vi "Read Voltage.vi"(8 "error in":errorcluster, 11 "Voltmeter CFG in":refnum<class "Voltmeter CFG.lvclass">) -> (0 "error out":errorcluster, 2 "Voltage":dbl format="%#_g V", 3 "Voltmeter CFG out":refnum<class "Voltmeter CFG.lvclass">)   [LabVIEW 2023, in "OWON SDS1022.lvlib" / "Voltmeter CFG.lvclass"]
uses:
  Voltmeter CFG.lvclass
  HAL/Scope VISA/Configuration/Scope VISA CFG.lvclass/Scope VISA CFG.ctl
  Voltmeter CFG.lvclass/Voltmeter CFG.ctl
  <vilib>/Analysis/baseanly.llb/Mean (DBL).vi
  <vilib>/Analysis/NI_AALBase.lvlib
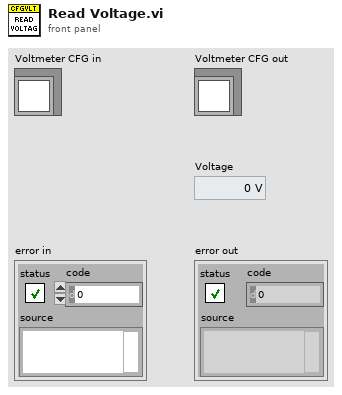
[diagram p1: front panel]
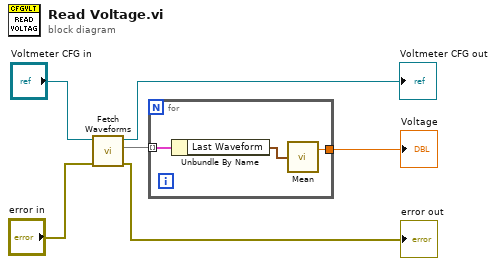
[diagram p0: block diagram]
diagram:
  n1 = call-dynamic "Fetch Waveforms.vi"("error in"="error in", "Fetch Display CFG in"="Voltmeter CFG in") -> ("error out"=→"error out":errorcluster, "Last Waveforms"=w3:map{u8, waveform(dbl)}, "Fetch Display out"=→"Voltmeter CFG out":refnum<class "Voltmeter CFG.lvclass">)  [unwired: 7 in]
  n2 = for {
    tunnel: w3 -> [w8] mode=indexing
    tunnel: [w9] -> w2
    n3 = Unbundle By Name(w8) -> ("Last Waveform"=w7:waveform(dbl))
    n4 = call-poly <vilib>:"Mean.vi"("X"=w7) -> ("mean"=w9:dbl)  [unwired: 1 out]
  }
  "Voltage" <- w2
